vi "Helper SubVI - Signal Sweep (wa).vi"(7 "reset (F)":bool, 10 "shift (%)":dbl=25.0, 11 "Signal in":dbl[](array[numeric])) -> (3 "Signal out":dbl[](array[numeric]))   [LabVIEW 2023]
doc: "Rotates the signal or gets a subset from the input signal."
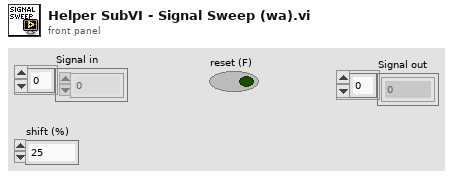
[diagram p1: front panel]
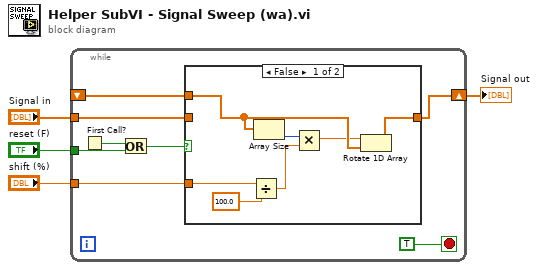
[diagram p0: block diagram]
diagram:
  n1 = while {
    shift-right: [w10] -> w4
    shift-left: _ -> [w8]
    tunnel: "reset (F)" -> [w7]
    tunnel: "Signal in" -> [w6]
    tunnel: "shift (%)" -> [w5]
    stop <- TRUE stop-if-true
    n2 = First Call?() -> (First Call?: T/F=w12:bool)
    n3 = Or(x=w12, y=w7) -> (x .or. y?=w11:bool)
    n4 = case shown="False" w11 {
      tunnel: w6 -> [_ w20]
      tunnel: [w18 w20] -> w10
      tunnel: w8 -> [w15 _]
      tunnel: w5 -> [w13 _]
      frame False {
        n5 = Divide(x=w13, y=100.0) -> (x/y=w17:dbl)
        n6 = Array Size(array=w15) -> (size(s)=w19:i32)
        n7 = Multiply(x=w19, y=w17) -> (x*y=w14:dbl)
        n8 = Rotate 1D Array(1:w15, 2:w14) -> (0:w18:dbl[])
      }
      frame True {
      }
    }
  }
  "Signal out" <- w4
